vi "calcCrcYldrm.vi"(1 "inpStr":string) -> (0 "crcVal":u8 format="%x")   [LabVIEW 2015]
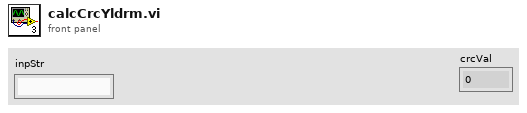
[diagram p1: front panel]
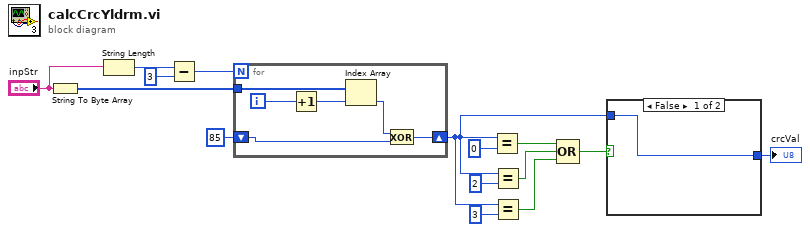
[diagram p0: block diagram]
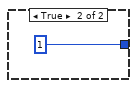
[diagram p2: hidden frame]
diagram:
  n1 = String To Byte Array(string="inpStr") -> (unsigned byte array=w15:u8[])
  n2 = String Length(string="inpStr") -> (length=w12:i32)
  n3 = Subtract(x=w12, y=3) -> (x-y=w10:i32)
  n4 = for {
    N: w10 -> [_]
    tunnel: w15 -> [w20]
    shift-right: [w17] -> w2
    shift-left: u8 85 -> [w16]
    i -> [w21]
    n5 = Increment(x=w21) -> (x+1=w19:i32)
    n6 = Index Array(array=w20, index=w19) -> (element=w18:u8)
    n7 = Exclusive Or(1:w16, 2:w18) -> (0:w17:u8)
  }
  n8 = Equal?(x=w2, y=u8 0) -> (x = y?=w6:bool)
  n9 = Equal?(x=w2, y=u8 2) -> (x = y?=w5:bool)
  n10 = Equal?(x=w2, y=u8 3) -> (x = y?=w4:bool)
  n11 = Compound Arithmetic op=OR(w6, w5, w4) -> (w3:bool)
  n12 = case shown="False" w3 {
    tunnel: [w22 u8 1 ("y")] -> w1
    tunnel: w2 -> [w22 _]
    frame False {
    }
    frame True {
    }
  }
  "crcVal" <- w1
